vi "mastercontrol.vi"() -> ()   [LabVIEW 2022 SP3]
uses:
  Motion Controllers/NI_controller/-NI_MotionRoutines/MotionSys.ctl
  -ScanSystem/Controls/location.ctl
  Digitizers/-DigitizerRoutines/DigConfig.ctl
  Pulsers/pulser.ctl
  Switch Modules/SwitchOption.ctl
  -ScanSystem/Controls/EKG_Mode.ctl
  Digitizers/-DigitizerRoutines/Digitizer.ctl
  -ScanSystem/Controls/Breath_Mode.ctl
  Spectrometers/OceanOptics/OceanOpticsVIs.llb/SpectrometerType.ctl
  Motion Controllers/-MotionRoutines/MotionGlobals.vi
  Digitizers/-DigitizerRoutines/DigitizerGlobals.vi
  Switch Modules/SwitchGlobals.vi
  Pulsers/PulserGlobals.vi
  <instrlib>/niSwitch/niSwitch.llb/niSwitch Topologies.ctl
  <instrlib>/Newport ESP301/Newport ESP301.lvlib
  <instrlib>/LeCroy Wave Series/LeCroy Wave Series.lvlib
panel:
  in  "Debug Mode?":bool
  in  "Microscopy Scope":refnum<visa-resource-name>="USB0::0x05FF::0x1023::4607N02183::INSTR"
  in  "Initial Setup\nComplete":bool
  in  "Bypass 2nd\nDigi Init":bool
  in  "Breath Trig":T1 items=["Respir Trig Off", "Respir Ring1 (Ch1)", "Respir Ch0", "Dig Edge"]
  in  "Main Digitizer":T2=enum."NI Digitizer"
  in  "EKG Gate":T3 items=["Retro/Prosp Off", "Prosp Ext EKG", "Prosp IQ EKG", "Retro EKG", "Retro IQ", "Retro No EKG"]
  in  "Switch Unit":T4=enum."No Switch"
  in  "Pulser":T5=enum."No Pulser"
  in  "Digitizer Config":T6
  in  "Location":T7
  in  "LeCroy IP Address":refnum<visa-resource-name>="VICP::169.254.24.19"
  in  "Main Spectrometer":T8 items=["No Spectrometer", "Ocean QE_Pro"]
  in  "Select V&A":bool
  in  "Motion System":T9=enum."Galil"
  in  "Start Scan":bool
  in  "Move to Home":bool
  in  "Man Cont":bool
  in  "NI Cards":i32=3
  in  "Therapy":bool
  in  "ExitSendCmd":bool
  # "Motion"
  # "No NI Motion Support!!!!!!!!\nOnly works with 64bit LV."
  # "SCAN"
  # "© 2022\nWeill Cornell"
  # "Options"
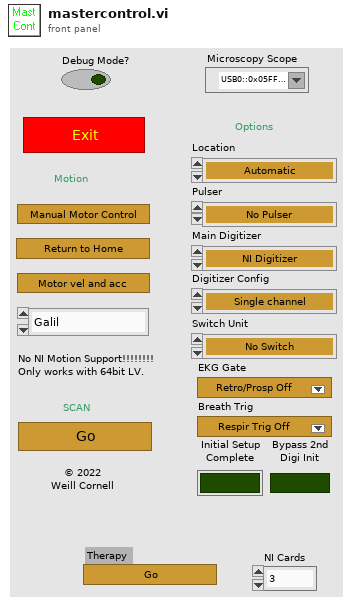
[diagram p1: front panel]
types:
  T1 = typedef "Breath_Mode.ctl" = u16
  T2 = typedef "Digitizer.ctl" = enum16{"Acqiris Digitizer", "NI Digitizer", "LeCroy", "GaGe", "AlazarTech", "No Digitizer", "Teledyne"}
  T3 = typedef "EKG_Mode.ctl" = u16
  T4 = typedef "SwitchOption.ctl" = enum16{"Cytex", "Pickering", "NI Switch", "No Switch", "Riverside USB"}
  T5 = typedef "pulser.ctl" = enum16{"Pan 5900", "Daxsonics", "Agilent 33xxx", "UTEX", "JSR", "WMC Mono-Cycle", "No Pulser", "NYU AVTECH", "Tabor W1281A", "Pan 5800", "Unlisted", "Tabor WX2182B"}
  T6 = typedef "DigConfig.ctl" = enum16{"Single channel", "2 Chans w/ 2 Acqiris", "2 Chans w/ 1 Acqiris", "5-CH Pulser New", "5-CH pulser w/ ann array", "5-pass style ann array", "Empty"}
  T7 = typedef "location.ctl" = enum16{"Automatic", "WCM Main", "Hawaii", "Columbia MM3000", "Columbia  NI System", "NYU", "RRI 2", "UHI Allen", "CUMC RT", "Chiba", "Stony Brook", "WCM Microscopy", "WCM Aeoretch", "WCM Optics Lab", "WCM Main 2Axis", "WCM Rotation", "WCM SAM SMAC", "SERI GP"}
  T8 = typedef "SpectrometerType.ctl" = u16
  T9 = typedef "MotionSys.ctl" = enum16{"MM3000", "NI 735x", "Newport ESP", "No Motion Card", "Galil"}
  T10 = typedef "DigitizerSettings.ctl" = cluster{"Digitizer delay (us) ":dbl, "rf points per line":i32, "lines per plane":i32, "Samp Rate (Hz)":dbl, "Additional dig delay (us)":dbl, "Voltage Scale":dbl, "Pre-Looks":i32, "Offset delay (us)":dbl, "bits A/D":i8, "Avg Num":i32, "DigTimeOut":sgl, "Rel Dig Delay":sgl, "Dig Ch":i32, "LeCroyCluster":cluster{"LeCroy Channels":bool[], "LC read pt offset":dbl, "Sweep Avg":bool}, "Main Digitizer":T2, "Dig Config":T6, "Digitizer ID Cluster":T11, "Trigger Settings":cluster{"Trig Source":u16, "Trig Coupling":u16, "Trig Slope":u16, "Level (mV)":dbl}, "Bulk Acq":bool, "Bulk Start Indexes":i32[], "Data Ref RF":refnum<data-value>, "NI ID/Channel":cluster{"NI ID":refnum<k15>, "NI CH":i32}[], "Total Dig CH":i32, "Xtra Ann Trig delay (us)":dbl, "Fix Z Delay?":bool, "One Way Transmission?":bool, "Data Ref Log":refnum<data-value>}
  T11 = typedef "DigitizerID.ctl" = cluster{"Acqiris/Alazar/SP ID":u32[], "NI Instr Handles":refnum<k15>[], "LeCroy VISA":refnum<visa-resource-name>, "GaGe Handle":cluster{"Handle":u32, "Sample size":u32, "Resolution":i32, "Offset":i32, "Channels":u32, "Boards":u32}, "ATS Ref":string, "Acqiris Address":string[], "ADQRef":refnum<k24>, "adq_cu_ptr":refnum<k24>}
  T12 = typedef "MotionParameters.ctl" = cluster{"No Motion?":bool, "Motion System":T9, "Motion Bd ID":u8, "Motion Profile":string, "# Axis":i8, "Reverse Z axis?":bool, "SMAC Axis":u16, "scan pair":T13, "RT fps":sgl, "Steps per mm":i32[], "Motor Parameters":cluster{"velocity ct/s":dbl[], "accel ct/s^2":dbl[]}, "One Way Scan":bool, "Reverse One Way Scan":bool, "Global Position (mm)":dbl[], "Plane":i32, "Distance between\nscan lines (um)":sgl, "Distance between\nscan planes (um)":sgl, "number of scan planes":i32, "Total steps in line":i32, "Xtra plane\ndistance  (um)":i32, "Xtra planes ":i32, "Add Axis":bool, "overshoot cts":i32, "BKPT Shift":i32, "Scan Start Time (ms)":u32, "ESP VISA":refnum<visa-resource-name>, "3rd Axis":T14, "GL Ref Out":refnum<k7>, "Galil Address":string}
  T13 = typedef "ScanAxis.ctl" = enum16{"y-(x) scan", "x-(y) scan", "z-(x) scan", "z-(y) scan", "y-(z) scan", "x-(z) scan", "w-(x) scan", "w-(y) scan", "w-(z) scan", "x-(w) scan", "y-(w) scan", "z-(w) scan"}
  T14 = typedef "3rdAxis.ctl" = u16
  T15 = enum8{"Enabled", "Disabled", "Disabled and Grayed Out"}
  T16 = enum16{"Absolute Position", "Relative Position", "Velocity", "Relative to Cap Pos", "Modulus Position", "Absolute Contouring", "Relative Contouring"}
  T17 = typedef "niSwitch Topologies.ctl" = string
  T18 = cluster{"Pulser":refnum<vi>, "Switch Unit":refnum<vi>, "Main Digitizer":refnum<vi>, "Digitizer Config":refnum<vi>, "EKG Gate":refnum<vi>, "Breath Trig":refnum<vi>, "Motion System":refnum<vi>, " LeCroy IP Address":refnum<vi>, "Main Spectrometer":refnum<vi>}
  T19 = typedef "Dual XDCR Complete Settings.ctl" = cluster{"Scan Size":dbl[], "XDCR Offset":dbl[], "Found Home":bool, "XDCR Settings":T20[]}
  T20 = typedef "XDCRSettings.ctl" = cluster{"Transducer Name":string, "Motion Settings":cluster{"Distance between\nscan lines (um)":sgl, "Distance between\nscan planes (um)":sgl}, "Digitizer Settings":cluster{"RF data Sampling":cluster{"Sampling Rate":dbl, "Ref Delay (ms)":dbl, "rf points per line":i32}, "Time scale per Div":dbl, "Voltage Scale":dbl, "Additional dig delay (ms)":dbl}, "Filter Prams":cluster{"low cutoff":i32, "order":i32, "high cutoff":i32}, "XDCR Focal Length":dbl, "Data Vertical Center":dbl, "Image Vertical Offset":dbl, "Daxsonics Settings":T21, "Panametrics Settings":T22, "JSR Complete":T23, "UT340 Controls":T38}
  T21 = typedef "Dax_Control_Cluster.ctl" = cluster{"Freq (MHz) ":u16, "Voltage (V)":u16, "Gain (dB)":u16}
  T22 = typedef "Pana5900.ctl" = cluster{"ENERGY (uJ)":u16, "DAMPING (Ohm)":u16, "HP FILT (KHz) ":u16, "LP FILT (MHz)":u16, "MODE":u16, "PRF (KHz)":u16, "GAIN (db)":u16, "COARSE ATTENUATION":u16, "FINE ATTENUATION":u16}
  T23 = typedef "JSR Complete.ctl" = cluster{"JSR Pulse Settings":T24, "JSR Receive Settings":T29, "JSR Trigger Settings":T34}
  T24 = typedef "JSR Pulse.ctl" = cluster{"Damping":T25, "Pulse Energy Level":T26, "Pulser Impedance":T27, "Pulser Voltage (V)":T28}
  T25 = typedef "Damping.ctl" = i16
  T26 = typedef "Energy.ctl" = u16
  T27 = typedef "Z.ctl" = u16
  T28 = typedef "Volt.ctl" = i16
  T29 = typedef "JSR Recieve.ctl" = cluster{"Receiver Mode":T30, "High Pass Filter":T31, "Low Pass Filter":T32, "Gain (dB)":T33}
  T30 = typedef "Mode.ctl" = i8
  T31 = typedef "HPF.ctl" = u16
  T32 = typedef "LPF.ctl" = u16
  T33 = typedef "Gain.ctl" = i8
  T34 = typedef "JSR Trigger.ctl" = cluster{"External Trigger Limit":T35, "Trigger Source":T36, "PRF (Hz)":T37}
  T35 = typedef "Trig Limit.ctl" = i8
  T36 = typedef "Trig Source.ctl" = i8
  T37 = typedef "PRF.ctl" = dbl
  T38 = typedef "UTEX Controls.ctl" = cluster{"High Pass On":bool, "High Pass Filter (MHz)":i16, "Low Pass On":bool, "Low Pass Filter (MHz)":i16, "PE Gain (dB)":i16, "Voltage":i16, "Pulse Width (ns)":dbl, "Mode":bool, "PC Gain (dB)":i16, "Trig Source":bool, "Rep Rate (Hz)":i16, "PULSE":bool}
  T39 = cluster{"Therapy frequency (MHz)":dbl, "Therapy amplitude (mV)":dbl, "time therapy on (s)":dbl, "Therapy Delay (ms) ":dbl, "Time (s)":dbl}
  T40 = cluster{"Handle":u32, "Sample size":u32, "Resolution":i32, "Offset":i32, "Channels":u32, "Boards":u32}
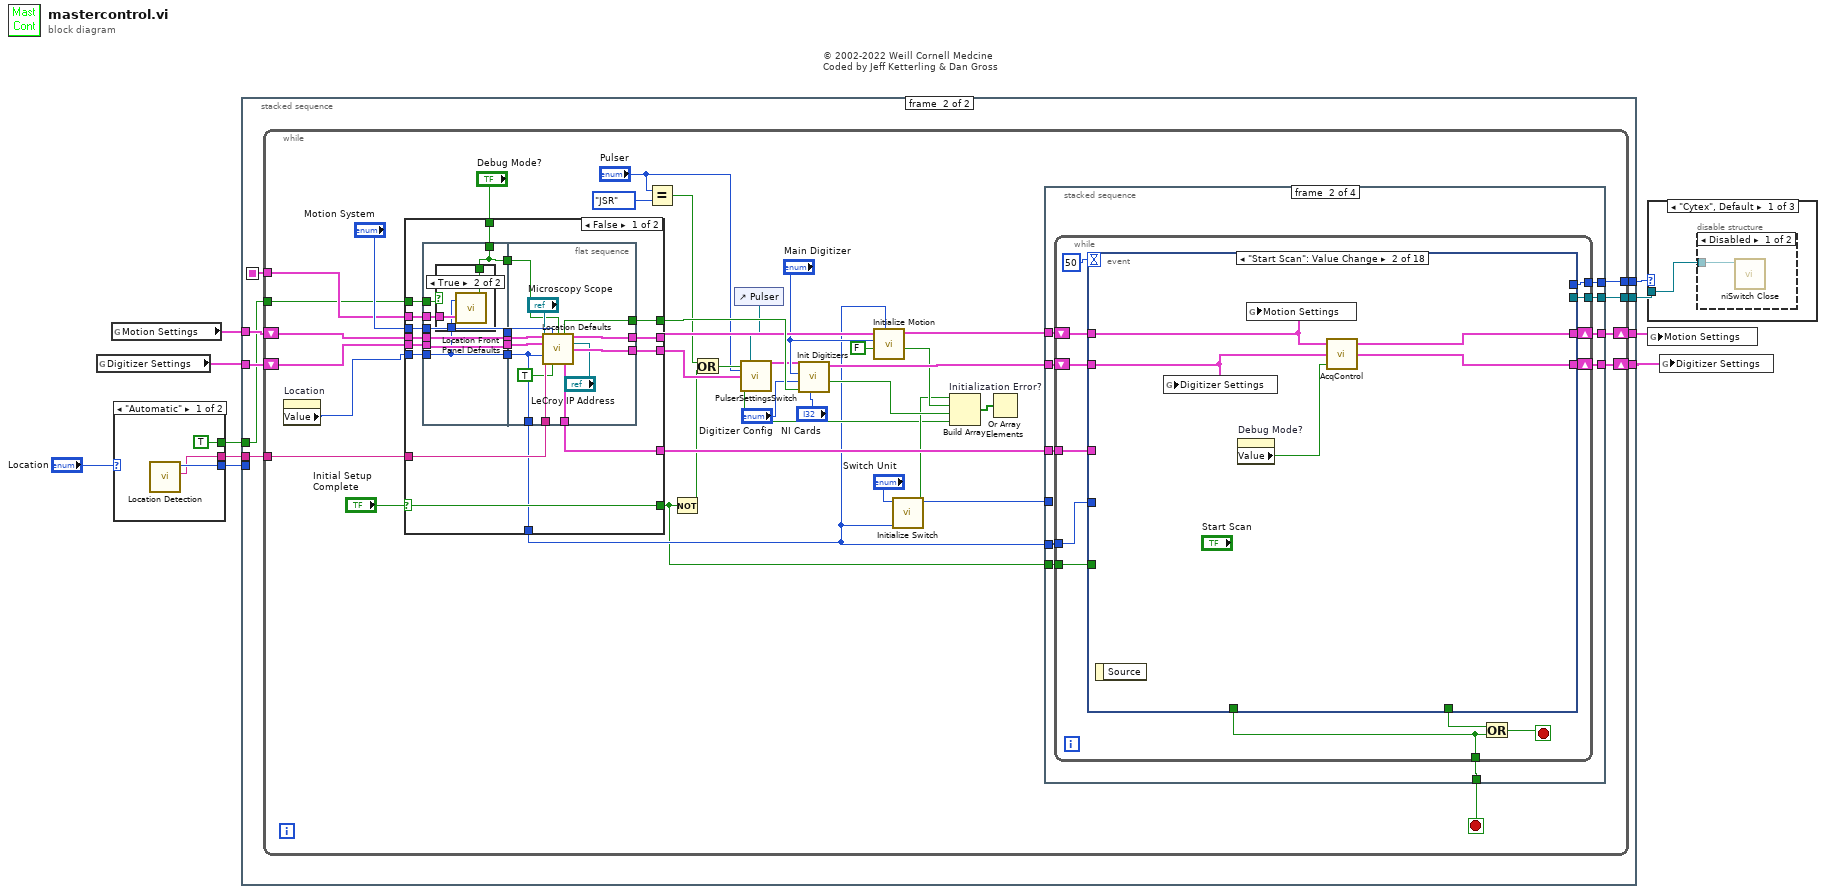
[diagram p0: block diagram]
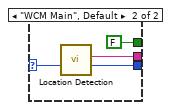
[diagram p2: hidden frame]
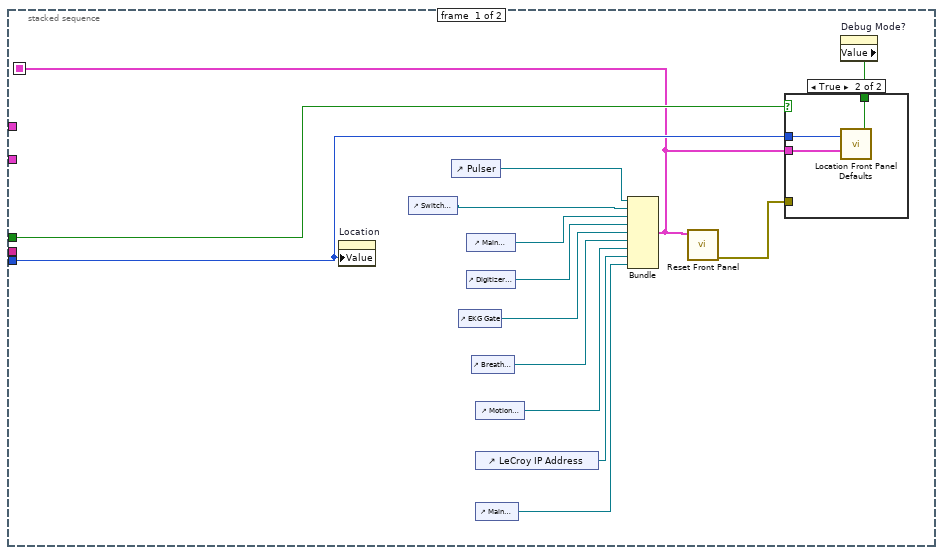
[diagram p3: hidden frame]
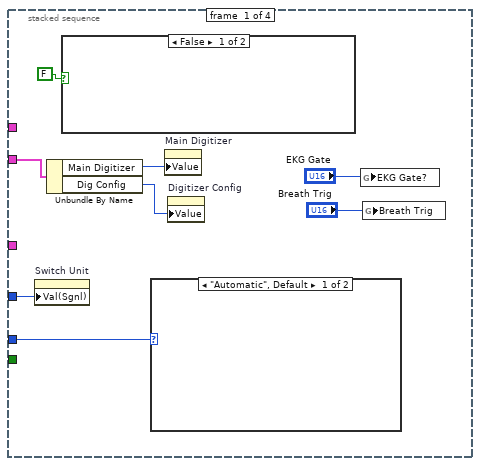
[diagram p5: hidden frame]
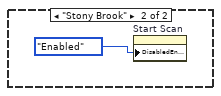
[diagram p6: hidden frame]
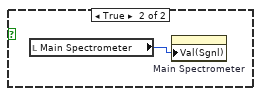
[diagram p7: hidden frame]
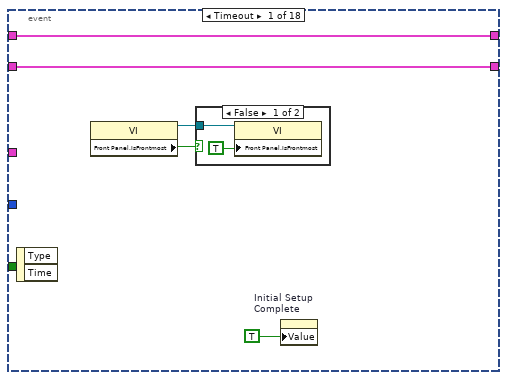
[diagram p8: hidden frame]
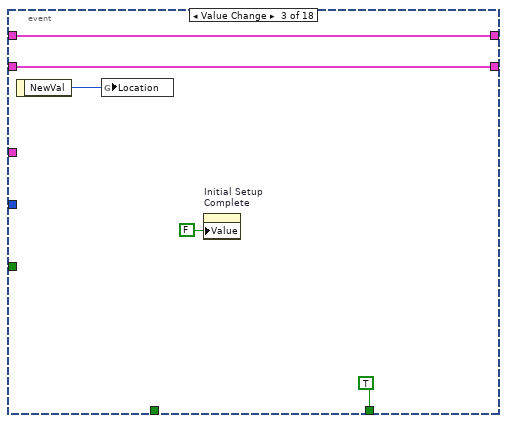
[diagram p10: hidden frame]
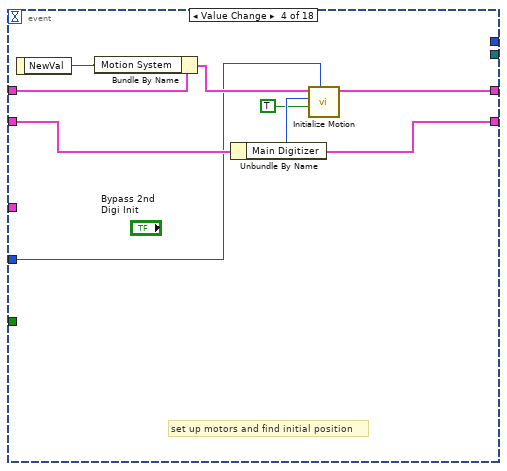
[diagram p11: hidden frame]
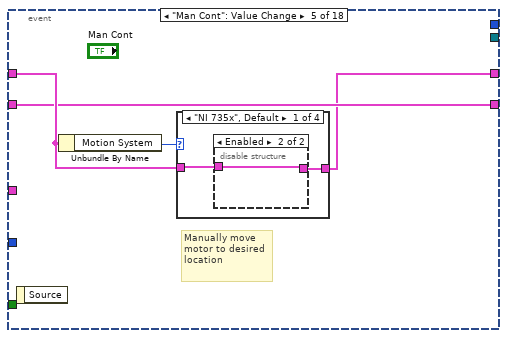
[diagram p12: hidden frame]
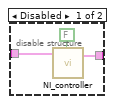
[diagram p13: hidden frame]
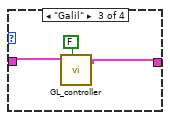
[diagram p15: hidden frame]
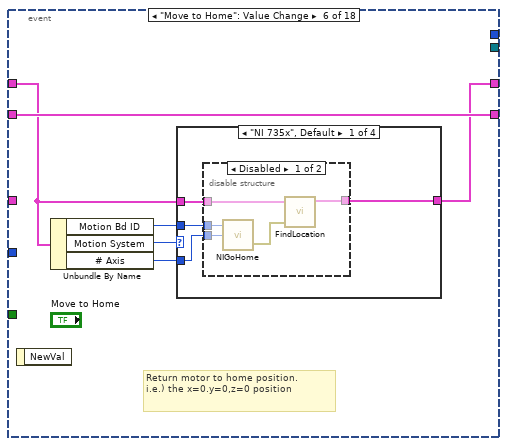
[diagram p17: hidden frame]
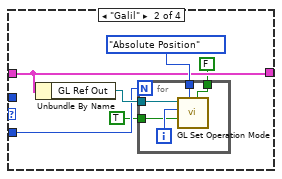
[diagram p19: hidden frame]
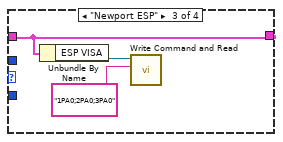
[diagram p20: hidden frame]
diagram:
  # "© 2002-2022 Weill Cornell Medcine\nCoded by Jeff Ketterling & Dan Gross"
  n1 = global read "DigitizerGlobals.vi" "Digitizer Settings"() -> (w6:T10)
  n2 = global read "MotionGlobals.vi" "Motion Settings"() -> (w7:T12)
  n3 = case shown="\"Automatic\"" "Location" {
    selector: "Location" -> [_ w16]
    tunnel: [w13 w16] -> w3
    tunnel: [w12 w14] -> w2
    tunnel: [TRUE ("Load Defaults") FALSE ("Load Defaults")] -> w1
    frame "Automatic" {
      n4 = call "Location Detection.vi"() -> ("Computer Name"=w12:string, "Location"=w13:T7)  [unwired: 10 in]
    }
    frame "WCM Main", Default {
      n5 = call "Location Detection.vi"() -> ("Computer Name"=w14:string)  [unwired: 10 in, 1 out]
    }
  }
  n6 = stacked-sequence {
    seq-local: [w18 _] -> [_ w36]
    tunnel: [_ w42] -> w10
    tunnel: [_ w41] -> w9
    tunnel: [_ w40] -> w5
    tunnel: w6 -> [_ w39]
    tunnel: w7 -> [_ w38]
    tunnel: [_ w37] -> w8
    tunnel: w3 -> [w25 _]
    tunnel: w2 -> [_ w35]
    tunnel: w1 -> [w24 w34]
    frame #0 {
      n7 = property on="Location" class="Enum (strict)"("Value"=w25) -> ()  [unwired: 2 in, 2 out]
      n8 = control-ref of="Switch Unit"() -> (w17:refnum<vi>)
      n9 = control-ref of="Pulser"() -> (w19:refnum<vi>)
      n10 = control-ref of="EKG Gate"() -> (w29:refnum<vi>)
      n11 = control-ref of="Main Digitizer"() -> (w22:refnum<vi>)
      n12 = control-ref of="Digitizer Config"() -> (w23:refnum<vi>)
      n13 = control-ref of="Breath Trig"() -> (w28:refnum<vi>)
      n14 = control-ref of="Motion System"() -> (w27:refnum<vi>)
      n15 = control-ref of="LeCroy IP Address"() -> (w26:refnum<vi>)
      n16 = control-ref of="Main Spectrometer"() -> (w30:refnum<vi>)
      n17 = Bundle("Pulser"=w19, "Switch Unit"=w17, "Main Digitizer"=w22, "Digitizer Config"=w23, "EKG Gate"=w29, "Breath Trig"=w28, "Motion System"=w27, "LeCroy IP Address"=w26, "Main Spectrometer"=w30) -> (w18:T18)  [unwired: 1 in]
      n18 = call "Reset Front Panel.vi"("output cluster"=w18) -> ("error out"=w20:errorcluster)  [unwired: 10 in]
      n19 = property on="Debug Mode?" class="Bool (strict)"() -> ("Value"=w21:bool)  [unwired: 2 in, 2 out]
      n20 = case shown="True" w24 {
        tunnel: w18 -> [_ w32]
        tunnel: w25 -> [_ w33]
        tunnel: w21 -> [_ w31]
        tunnel: w20 -> [_ _]
        frame False {
        }
        frame True {
          n21 = call "Location Front Panel Defaults.vi"("Debug Mode?"=w31, "output cluster"=w32, "Location"=w33) -> ()
        }
      }
    }
    frame #1 {
      n22 = while {
        tunnel: [w81] -> w42
        tunnel: [w80] -> w41
        shift-right: [w79] -> w40
        shift-left: w39 -> [w76]
        shift-right: [w78] -> w37
        shift-left: w38 -> [w77]
        tunnel: w36 -> [w60]
        tunnel: w35 -> [w58]
        tunnel: w34 -> [w57]
        stop <- w82 stop-if-true
        n23 = property on="Location" class="Enum (strict)"() -> ("Value"=w43:T7)  [unwired: 2 in, 2 out]
        n24 = case shown="False" "Initial Setup\nComplete" {
          selector: "Initial Setup\nComplete" -> [w338 w381]
          tunnel: w77 -> [w353 w379]
          tunnel: [w352 w377] -> w70
          tunnel: w76 -> [w351 w384]
          tunnel: [w341 w384] -> w73
          tunnel: [w350 w383] -> w74
          tunnel: w43 -> [w347 w380]
          tunnel: [w349 w382] -> w75
          tunnel: "Motion System" -> [w348 w378]
          tunnel: w60 -> [w342 _]
          tunnel: w58 -> [w340 _]
          tunnel: w57 -> [w339 _]
          tunnel: [w338 w381] -> w44
          tunnel: "Debug Mode?" -> [w337 _]
          tunnel: [w336 w380] -> w45
          frame False {
            n25 = flat-sequence {
              tunnel: w347 -> [w356]
              tunnel: w348 -> [w358]
              tunnel: w351 -> [w359]
              tunnel: w353 -> [w360]
              tunnel: [w360] -> w346
              tunnel: [w359] -> w345
              tunnel: [w358] -> w344
              tunnel: [w356] -> w343
              tunnel: w342 -> [w357]
              tunnel: w339 -> [w355]
              tunnel: w337 -> [w354]
              tunnel: [w354] -> w335
              tunnel: [w375] -> w352
              tunnel: [w370] -> w350
              tunnel: [w373] -> w349
              tunnel: w346 -> [w376]
              tunnel: w345 -> [w374]
              tunnel: w344 -> [w372]
              tunnel: w343 -> [w366]
              tunnel: [w371] -> w341
              tunnel: w340 -> [w369]
              tunnel: [w366] -> w336
              tunnel: w335 -> [w364]
              frame #0 {
                n26 = case shown="True" w355 {
                  tunnel: w357 -> [_ w363]
                  tunnel: w356 -> [_ w361]
                  tunnel: w354 -> [_ w362]
                  frame False {
                  }
                  frame True {
                    n27 = call "Location Front Panel Defaults.vi"("Debug Mode?"=w362, "output cluster"=w363, "Location"=w361) -> ()
                  }
                }
              }
              frame #1 {
                n28 = call "Location Defaults.vi"("Motion Settings In"=w376, "Motion System"=w372, "Debug Mode?"=w364, "Digitizer Settings In"=w374, "LeCroy IP Address"="LeCroy IP Address", "Microscopy Scope"="Microscopy Scope", "Location In"=w366, "Computer Name"=w369, "Create Data Folder"=TRUE) -> ("Bypass 2nd dig init"=w370:bool, "Motion Settings"=w375:T12, "Digitizer Settings"=w371:T10, "Dual XDCR Settings"=w373:T19)  [unwired: 1 in, 2 out]
              }
            }
          }
          frame True {
            n29 = global read "SwitchGlobals.vi" "Dual XDCR Settings"() -> (w382:T19)
            n30 = Bundle By Name(cluster=w379, "Motion System"=w378) -> (w377:T12)
            n31 = property on="Bypass 2nd\nDigi Init" class="Bool (strict)"() -> ("Value"=w383:bool)  [unwired: 2 in, 2 out]
          }
        }
        n32 = Equal?(x="Pulser", y=pulser."JSR") -> (x = y?=w48:bool)
        n33 = Not(x=w44) -> (.not. x?=w47:bool)
        n34 = Or(x=w48, y=w47) -> (x .or. y?=w51:bool)
        n35 = control-ref of="Pulser"() -> (w46:refnum<vi>)
        n36 = call "PulserSettingsSwitch.vi"("Initilize?"=w51, "Pulser Ref"=w46, "Pulser"="Pulser", "Digitizer Settings in"=w73) -> ("Digitizer Settings out"=w55:T10, "Initialization Failed!!"=w54:bool)  [unwired: 9 in, 1 out]
        n37 = call "Init Digitizers.vi"("NI Cards"="NI Cards", "Bypass 2nd Digitizer Init"=w74, "Digitizer Config"="Digitizer Config", "Main Digitizer"="Main Digitizer", "Digitizer Settings in"=w55) -> ("Initialization Failed!!"=w65:bool, "Digitizer Settings"=w68:T10)  [unwired: 4 in, 1 out]
        n38 = call "Initialize Motion.vi"("Location"=w45, "Bypass Motion Init"=FALSE, "Main Digitizer"="Main Digitizer", "Motion Settings In"=w70) -> ("Initialization Failed!!"=w66:bool, "Motion Settings"=w69:T12)  [unwired: 5 in, 1 out]
        n39 = call "Initialize Switch.vi"("Location"=w45, "Switch Unit In"="Switch Unit") -> ("Initialization Failed!!"=w62:bool, "Switch Unit"=w63:T4)  [unwired: 8 in]
        n40 = Build Array "Initialization Error?"(w62, w66, w65, w54) -> (w67:bool[])
        n41 = Or Array Elements(Boolean array=w67) -> ()  [unwired: 1 out]
        n42 = stacked-sequence {
          tunnel: [_ w98 _ _] -> w80
          tunnel: [_ w97 _ _] -> w81
          tunnel: [_ w93 _ _] -> w82
          tunnel: w68 -> [w86 w96 _ w302]
          tunnel: [_ w102 _ _] -> w79
          tunnel: w69 -> [_ w99 _ w303]
          tunnel: [_ w101 _ _] -> w78
          tunnel: w75 -> [_ w100 _ _]
          tunnel: w63 -> [w87 _ _ _]
          tunnel: w45 -> [w83 w95 _ _]
          tunnel: w44 -> [_ w94 _ _]
          frame #0 {
            n43 = property on="Switch Unit" class="Enum (strict)"("Val(Sgnl)"=w87) -> ()  [unwired: 2 in, 2 out]
            n44 = Unbundle By Name(w86) -> ("Main Digitizer"=w85:T2, "Dig Config"=w84:T6)
            n45 = case shown="False" FALSE {
              frame False {
              }
              frame True {
                n46 = local read "Main Spectrometer"() -> (w92:T8)
                n47 = property on="Main Spectrometer" class="Ring (strict)"("Val(Sgnl)"=w92) -> ()  [unwired: 2 in, 2 out]
              }
            }
            n48 = case shown="\"Automatic\", Default" w83 {
              frame "Automatic", Default {
              }
              frame "Stony Brook" {
                n49 = property on="Start Scan" class="Bool"("DisabledEnum"=T15."Enabled" ("Disabled")) -> ()  [unwired: 2 in, 2 out]
              }
            }
            n50 = property on="Main Digitizer" class="Enum (strict)"("Value"=w85) -> ()  [unwired: 2 in, 2 out]
            n51 = property on="Digitizer Config" class="Enum (strict)"("Value"=w84) -> ()  [unwired: 2 in, 2 out]
            n52 = global write "MotionGlobals.vi" "EKG Gate?"("EKG Gate") -> ()
            n53 = global write "MotionGlobals.vi" "Breath Trig"("Breath Trig") -> ()
          }
          frame #1 {
            n54 = while {
              shift-right: [w111] -> w102
              shift-left: w96 -> [w112]
              shift-right: [w109] -> w101
              shift-left: w99 -> [w110]
              tunnel: w100 -> [w108]
              tunnel: [w107] -> w98
              tunnel: [w106] -> w97
              tunnel: w95 -> [w105]
              tunnel: w94 -> [w104]
              tunnel: [w103] -> w93
              stop <- w114 stop-if-true
              n55 = event shown="[1] \"Start Scan\": Value Change" {
                selector: _ -> [_ _ _ _ _ _ _ _ _ _ _ _ _ _ _ _ _ _]
                dyn-events: _ -> [_ _ _ _ _ _ _ _ _ _ _ _ _ _ _ _ _ _]
                timeout: 50 -> [_ _ _ _ _ _ _ _ _ _ _ _ _ _ _ _ _ _]
                tunnel: [_ _ TRUE _ _ _ _ _ _ TRUE TRUE TRUE TRUE _ _ TRUE _ _] -> w113
                tunnel: w112 -> [w120 w124 w131 w136 w142 w162 w191 w210 w248 w255 w261 w264 w268 w270 w273 w279 w286 w288]
                tunnel: [w120 w125 w131 w136 w142 w162 w191 w208 w248 w254 w261 w264 w268 w270 w273 w278 w286 w288] -> w111
                tunnel: w110 -> [w119 w127 w130 w138 w143 w159 w189 w209 w247 w252 w260 w263 w267 w269 w272 w276 w285 w287]
                tunnel: [w119 w126 w130 w139 w141 w157 w188 w207 w247 w252 w260 w263 w267 w269 w272 w276 w285 w287] -> w109
                tunnel: w108 -> [_ _ _ _ _ _ _ w206 _ _ _ _ _ _ _ _ _ _]
                tunnel: [_ _ _ _ _ _ _ w205 _ _ _ _ _ _ _ _ _ _] -> w107
                tunnel: [_ _ _ _ _ _ _ w203 _ _ _ _ _ _ _ _ _ _] -> w106
                tunnel: w105 -> [_ _ _ w133 _ _ w187 w204 _ _ _ _ _ _ _ _ _ _]
                tunnel: w104 -> [_ _ _ _ _ _ _ w202 _ _ _ _ _ _ _ _ _ _]
                tunnel: [_ _ _ _ _ _ _ _ "ExitSendCmd" _ _ _ _ _ _ _ _ _] -> w103
                event Timeout {
                  n56 = event-data() -> ()  [unwired: 3 out]
                  n57 = property class="VI"() -> (reference out=w118:refnum<vi>, "Front Panel.IsFrontmost"=w117:bool)  [unwired: 2 in, 1 out]
                  n58 = case shown="False" w117 {
                    tunnel: w118 -> [w122 _]
                    frame False {
                      n59 = property class="VI"(reference=w122, "Front Panel.IsFrontmost"=TRUE) -> ()  [unwired: 1 in, 2 out]
                    }
                    frame True {
                    }
                  }
                  n60 = property on="Initial Setup\nComplete" class="Bool (strict)"("Value"=TRUE ("Initial Setup\nComplete")) -> ()  [unwired: 2 in, 2 out]
                }
                event "Start Scan": Value Change {
                  n61 = event-data() -> ()  [unwired: 2 out]
                  n62 = global write "DigitizerGlobals.vi" "Digitizer Settings"(w124) -> ()
                  n63 = property on="Debug Mode?" class="Bool (strict)"() -> ("Value"=w123:bool)  [unwired: 2 in, 2 out]
                  n64 = global write "MotionGlobals.vi" "Motion Settings"(w127) -> ()
                  n65 = call "AcqControl.vi"("Debug Mode?"=w123, "Digitizer Settings"=w124, "Motion Settings In"=w127) -> ("Digitizer Settings Out"=w125:T10, "Motion Settings Out"=w126:T12)  [unwired: 1 in]
                }
                event Value Change {
                  n66 = event-data() -> ("NewVal"=w129:T7)  [unwired: 1 out]
                  n67 = global write "MotionGlobals.vi" "Location"(w129) -> ()
                  n68 = property on="Initial Setup\nComplete" class="Bool (strict)"("Value"=FALSE ("Initial Setup\nComplete")) -> ()  [unwired: 2 in, 2 out]
                }
                event Value Change {
                  # "set up motors and find initial position"
                  n69 = event-data() -> ("NewVal"=w140:T9)  [unwired: 1 out]
                  n70 = Bundle By Name(cluster=w138, "Motion System"=w140) -> (w137:T12)
                  n71 = Unbundle By Name(w136) -> ("Main Digitizer"=w135:T2)
                  n72 = call "Initialize Motion.vi"("Location"=w133, "Bypass Motion Init"=TRUE, "Main Digitizer"=w135, "Motion Settings In"=w137) -> ("Motion Settings"=w139:T12)  [unwired: 5 in, 2 out]
                }
                event "Man Cont": Value Change {
                  # "Manually move motor to desired\nlocation"
                  n73 = event-data() -> ()  [unwired: 2 out]
                  n74 = Unbundle By Name(w143) -> ("Motion System"=w144:T9)
                  n75 = case shown="\"NI 735x\", Default" w144 {
                    tunnel: w143 -> [w146 w152 w155 w156]
                    tunnel: [w145 w151 w154 w156] -> w141
                    frame "NI 735x", Default {
                      n76 = disable-structure shown="Enabled" {
                        disable-tunnel: w146 -> [w148 w150]
                        disable-tunnel: [w147 w150] -> w145
                        frame Disabled {
                          n77 = call "NI_controller.VI"("Motion Settings"=w148, "Initialize"=FALSE) -> ("Motion Settings Out"=w147:T12)  [unwired: 3 in, 1 out]
                        }
                        frame Enabled {
                        }
                      }
                    }
                    frame "Newport ESP" {
                      n78 = call "ESPControl.vi"("Motion Settings"=w152) -> ("Motion Settings Out"=w151:T12)  [unwired: 4 in, 1 out]
                    }
                    frame "Galil" {
                      n79 = call "GL_controller.VI"("Motion Settings"=w155, "Initialize"=FALSE) -> ("Motion Settings Out"=w154:T12)  [unwired: 3 in, 1 out]
                    }
                    frame "No Motion Card" {
                    }
                  }
                }
                event "Move to Home": Value Change {
                  # "Return motor to home position.\ni.e.) the x=0.y=0,z=0 position"
                  n80 = event-data() -> ()  [unwired: 2 out]
                  n81 = Unbundle By Name(w159) -> ("Motion Bd ID"=w161:u8, "Motion System"=w160:T9, "# Axis"=w158:i8)
                  n82 = case shown="\"NI 735x\", Default" w160 {
                    tunnel: w161 -> [w166 _ _ _]
                    tunnel: w159 -> [w164 w176 w183 w186]
                    tunnel: w158 -> [w165 w174 _ _]
                    tunnel: [w163 w176 w183 w186] -> w157
                    frame "NI 735x", Default {
                      n83 = disable-structure shown="Disabled" {
                        disable-tunnel: w166 -> [w171 _]
                        disable-tunnel: w165 -> [w170 _]
                        disable-tunnel: w164 -> [w168 _]
                        disable-tunnel: [w167 _] -> w163
                        frame Disabled {
                          n84 = call "NIGoHome.vi"("# Axis"=w170, "Board ID"=w171) -> ("error out"=w169:errorcluster)  [unwired: 1 in, 1 out]
                          n85 = call "FindLocation.vi"("Motion Settings"=w168, "error in (no error)"=w169) -> ("Motion Settings Out"=w167:T12)  [unwired: 1 in, 3 out]
                        }
                        frame Enabled {
                        }
                      }
                    }
                    frame "Galil" {
                      n86 = Unbundle By Name(w176) -> ("GL Ref Out"=w175:refnum<k7>)
                      n87 = for {
                        N: w174 -> [_]
                        tunnel: T16."Absolute Position" ("Position Mode (Absolute)") -> [w182]
                        tunnel: w175 -> [w181]
                        tunnel: TRUE ("Start Now?") -> [w179]
                        tunnel: FALSE ("LimitWarning?") -> [w178]
                        i -> [w180]
                        n88 = call "GL Set Operation Mode.vi"("LimitWarning?"=w178, "Position Mode (Absolute)"=w182, "Start Now?"=w179, "Axis"=w180, "Galil.IGalil"=w181) -> ()  [unwired: 4 in, 3 out]
                      }
                    }
                    frame "Newport ESP" {
                      n89 = Unbundle By Name(w183) -> ("ESP VISA"=w184:refnum<visa-resource-name>)
                      n90 = call <instrlib>:"Write Command and Read.vi"("Command"="1PA0;2PA0;3PA0", "VISA resource name"=w184) -> ()  [unwired: 5 in, 3 out]
                    }
                    frame "No Motion Card" {
                    }
                  }
                }
                event "Select V&A": Value Change {
                  # "Need to set global Motor Parameters\nto default for velocity and accel"
                  n91 = event-data() -> ()  [unwired: 2 out]
                  n92 = Unbundle By Name(w189) -> ("Motion System"=w190:T9)
                  n93 = case shown="\"NI 735x\", Default" w190 {
                    tunnel: w189 -> [w196 w198 w201]
                    tunnel: [w195 w199 w200] -> w188
                    tunnel: w187 -> [w194 _ _]
                    frame "NI 735x", Default {
                      n94 = call "UpdateVandAGlobals.vi"("Motion Settings"=w196) -> ("Motion Settings Out"=w195:T12)  [unwired: 3 in, 1 out]
                      n95 = call "Initialize_NI.vi"("Motion Settings"=w195, "Bypass Motion Init"=TRUE ("Bypass Init"), "Location"=w194) -> ()  [unwired: 2 in, 3 out]
                    }
                    frame "Galil" {
                      n96 = Unbundle By Name(w198) -> ("GL Ref Out"=w197:refnum<k7>)
                      n97 = call "GL_SetVandA.vi"("Motion Settings"=w198, "Refnum in"=w197) -> ("Motion Settings Out"=w199:T12)  [unwired: 7 in, 2 out]
                    }
                    frame "Newport ESP" {
                      n98 = call "UpdateVandAGlobals.vi"("Motion Settings"=w201) -> ("Motion Settings Out"=w200:T12)  [unwired: 3 in, 1 out]
                      n99 = call "Init ESP.vi"("Motion Settings In"=w200) -> ()  [unwired: 11 in]
                    }
                  }
                  n100 = local write "Select V&A"(FALSE) -> ()
                }
                event Value Change {
                  n101 = event-data() -> ("NewVal"=w203:T4)  [unwired: 1 out]
                  n102 = case shown="\"NI Switch\"" w203 {
                    tunnel: [_ w215 _ _] -> w205
                    tunnel: w209 -> [w211 w214 w221 w231]
                    tunnel: [w211 w214 w221 w228] -> w207
                    tunnel: w210 -> [w212 w213 w220 w230]
                    tunnel: [w212 w213 w220 w229] -> w208
                    tunnel: w206 -> [_ _ _ w224]
                    tunnel: w204 -> [_ _ _ w227]
                    tunnel: w202 -> [_ _ _ w226]
                    frame "Pickering" {
                    }
                    frame "NI Switch" {
                      n103 = disable-structure shown="Disabled" {
                        disable-tunnel: [w219 _] -> w215
                        frame Disabled {
                          n104 = call <instrlib>:"niSwitch Initialize With Topology.vi"("reset device (boolean value)"=TRUE, "topology name"=T17 "2593/16x1 Mux", "resource name"=refnum<k15> "NISwitch") -> ("instrument handle out"=w219:refnum<k15>)  [unwired: 7 in, 1 out]
                          n105 = global write "MotionGlobals.vi" "NI Switch"(w219) -> ()
                        }
                        frame Enabled {
                        }
                      }
                    }
                    frame "No Switch", Default {
                    }
                    frame "Riverside USB" {
                      n106 = Unbundle By Name(w224) -> ("XDCR Settings"=w223:T20[])
                      n107 = Array Size(array=w223) -> (size(s)=w225:i32)
                      n108 = Not Equal To 0?(x=w225) -> (x != 0?=w222:bool)
                      n109 = case shown="True" w222 {
                        tunnel: w231 -> [w233 w244]
                        tunnel: w230 -> [w232 w243]
                        tunnel: [w232 w242] -> w229
                        tunnel: w224 -> [_ w241]
                        tunnel: [w233 w239] -> w228
                        tunnel: w227 -> [_ w238]
                        tunnel: w226 -> [_ w236]
                        frame False {
                        }
                        frame True {
                          n110 = property on="Pulser" class="Enum (strict)"() -> ("Value"=w235:T5)  [unwired: 2 in, 2 out]
                          n111 = property on="Debug Mode?" class="Bool (strict)"() -> ("Value"=w234:bool)  [unwired: 2 in, 2 out]
                          n112 = call "SetupXDCRDefaults.vi"("Digitizer Settings in"=w243, "Pulser"=w235, "Debug Mode?"=w234, "Motion Settings in"=w244, "Dual XDCR Settings In"=w241, "Location"=w238, "Initial Setup Complete"=w236) -> ("Digitizer Settings out"=w242:T10, "Motion Settings out"=w240:T12, "Dual XDCR Settings"=w237:T19)  [unwired: 3 in, 3 out]
                          n113 = global write "SwitchGlobals.vi" "Dual XDCR Settings"(w237) -> ()
                          n114 = call "FindLocation.vi"("Motion Settings"=w240) -> ("Motion Settings Out"=w239:T12)  [unwired: 2 in, 3 out]
                        }
                      }
                    }
                  }
                  n115 = global write "SwitchGlobals.vi" "Switch Unit"(w203) -> ()
                }
                event "ExitSendCmd": Value Change {
                  n116 = event-data() -> ()  [unwired: 5 out]
                  n117 = property on="Pulser" class="Enum (strict)"() -> ("Value"=w246:T5)  [unwired: 2 in, 2 out]
                  n118 = case shown="\"Pan 5900\", Default" w246 {
                    frame "Pan 5900", Default {
                    }
                    frame "JSR" {
                      n119 = global read "PulserGlobals.vi" "JSR VISA"() -> (w250:refnum<visa-resource-name>)
                      n120 = property on="Initial Setup\nComplete" class="Bool (strict)"("Value"=FALSE ("Initial Setup\nComplete")) -> ()  [unwired: 2 in, 2 out]
                      n121 = call <instrlib>:"dpr300 Close.vi"("VISA resource name"=w250) -> ()  [unwired: 10 in, 1 out]
                    }
                  }
                }
                event Value Change {
                  n122 = event-data() -> ("NewVal"=w253:T6)  [unwired: 1 out]
                  n123 = Bundle By Name(cluster=w255, "Dig Config"=w253) -> (w254:T10)
                  n124 = property on="Initial Setup\nComplete" class="Bool (strict)"("Value"=FALSE ("Initial Setup\nComplete")) -> ()  [unwired: 2 in, 2 out]
                }
                event Value Change {
                  n125 = event-data() -> ("NewVal"=w259:T5)  [unwired: 1 out]
                  n126 = global write "PulserGlobals.vi" "Pulser"(w259) -> ()
                  n127 = property on="Initial Setup\nComplete" class="Bool (strict)"("Value"=FALSE ("Initial Setup\nComplete")) -> ()  [unwired: 2 in, 2 out]
                }
                event "Initial Setup\nComplete": Value Change {
                  n128 = event-data() -> ()  [unwired: 2 out]
                }
                event "Debug Mode?": Value Change {
                  n129 = event-data() -> ()  [unwired: 2 out]
                  n130 = property on="Initial Setup\nComplete" class="Bool (strict)"("Value"=FALSE ("Initial Setup\nComplete")) -> ()  [unwired: 2 in, 2 out]
                }
                event Value Change {
                  n131 = event-data() -> ("NewVal"=w271:T3)  [unwired: 1 out]
                  n132 = global write "MotionGlobals.vi" "EKG Gate?"(w271) -> ()
                }
                event Value Change {
                  n133 = event-data() -> ("NewVal"=w274:T1)  [unwired: 1 out]
                  n134 = global write "MotionGlobals.vi" "Breath Trig"(w274) -> ()
                }
                event Value Change {
                  n135 = event-data() -> ("NewVal"=w277:T2)  [unwired: 1 out]
                  n136 = Bundle By Name(cluster=w279, "Main Digitizer"=w277) -> (w278:T10)
                  n137 = property on="Initial Setup\nComplete" class="Bool (strict)"("Value"=FALSE ("Initial Setup\nComplete")) -> ()  [unwired: 2 in, 2 out]
                }
                event "Therapy": Value Change {
                  # "Therapy solo"
                  n138 = event-data() -> ()  [unwired: 2 out]
                  n139 = global read "PulserGlobals.vi" "Therapy Settings"() -> (w284:T39)
                  n140 = Unbundle By Name(w284) -> ("Therapy frequency (MHz)"=w283:dbl, "Therapy amplitude (mV)"=w282:dbl, "time therapy on (s)"=w281:dbl)
                  n141 = call "Therapy.vi"("Theraputic Freq (MHz)"=w283, "Time on"=w281, "Therapy amplitude (mV)"=w282) -> ()  [unwired: 3 in, 3 out]
                }
                event Value Change {
                  n142 = event-data() -> ("OldVal"=w289:T8, "NewVal"=w290:T8)  [unwired: 1 out]
                  n143 = global write "MotionGlobals.vi" "Main Spectrometer"(w290) -> ()
                  n144 = case shown="0, Default" w290 {
                    tunnel: w289 -> [w291 _]
                    frame 0, Default {
                      n145 = case shown="1" w291 {
                        tunnel: [_ w292] -> _
                        frame 0, Default {
                        }
                        frame 1 {
                          # "OceanLVClose"
                          n146 = global read "MotionGlobals.vi" "Ocean Wrapper"() -> (w292:u32)
                        }
                      }
                    }
                    frame 1 {
                      # "OceanLVInit"
                    }
                  }
                }
              }
              n147 = Or(x=w113, y=w103) -> (x .or. y?=w114:bool)
            }
          }
          frame #2 {
            # "Delete local temp files"
            n148 = global read "MotionGlobals.vi" "TempPath"() -> (w293:path)
            n149 = List Folder(path=w293) -> (path out=w295:path, filenames=w294:string[], error out=w296:errorcluster)  [unwired: 1 in, 3 out]
            n150 = case shown="No Error" w296 {
              tunnel: w295 -> [w298 _]
              tunnel: w294 -> [w297 _]
              frame No Error {
                n151 = for {
                  tunnel: w298 -> [w300]
                  tunnel: w297 -> [w299] mode=indexing
                  n152 = Build Path(base path=w300, name or relative path=w299) -> (appended path=w301:path)
                  n153 = Delete(path (use dialog)=w301) -> ()  [unwired: 1 in, 6 out]
                }
              }
              frame Error {
              }
            }
          }
          frame #3 {
            n154 = Unbundle By Name(w303) -> ("Motion System"=w304:T9, "# Axis"=w305:i8)
            n155 = Unbundle By Name(w302) -> ("Main Digitizer"=w306:T2)
            n156 = case shown="\"NI 735x\", Default" w304 {
              tunnel: w305 -> [_ w324 _]
              tunnel: w303 -> [_ w323 w334]
              frame "NI 735x", Default {
              }
              frame "Newport ESP" {
                n157 = Unbundle By Name(w323) -> ("ESP VISA"=w322:refnum<visa-resource-name>)
                n158 = for {
                  N: w324 -> [_]
                  tunnel: w322 -> [w329]
                  tunnel: [w328] -> w326
                  tunnel: [w327] -> w325
                  i -> [w331]
                  n159 = Increment(x=w331) -> (x+1=w332:i32)
                  n160 = call <instrlib>:"Enable Disable Motor.vi"("Action (OFF)"=FALSE, "Axis (1)"=w332, "VISA resource name"=w329) -> ("error out"=w327:errorcluster, "VISA resource name out"=w328:refnum<visa-resource-name>)  [unwired: 3 in]
                }
                n161 = call <instrlib>:"Close.vi"("error in (no error)"=w325, "VISA resource name"=w326) -> ()  [unwired: 9 in, 1 out]
              }
              frame "Galil" {
                n162 = Unbundle By Name(w334) -> ("GL Ref Out"=w333:refnum<k7>)
                n163 = Close Reference(reference=w333) -> ()  [unwired: 1 in, 1 out]
              }
            }
            n164 = case shown="\"NI Digitizer\"" w306 {
              tunnel: w302 -> [_ w310 w313 w318 _ w321]
              frame "Acqiris Digitizer", Default {
              }
              frame "NI Digitizer" {
                n165 = Unbundle By Name(w310) -> ("Digitizer ID Cluster.NI Instr Handles"=w309:refnum<k15>[])
                n166 = for {
                  tunnel: w309 -> [w311] mode=indexing
                  n167 = call <instrlib>:"niScope Close.vi"("instrument handle"=w311) -> ()  [unwired: 1 in, 14 out]
                }
              }
              frame "LeCroy" {
                n168 = Unbundle By Name(w313) -> ("Digitizer ID Cluster.LeCroy VISA"=w312:refnum<visa-resource-name>)
                n169 = call <instrlib>:"Write.vi"("Write Buffer"="VBS 'app.acquisition.Horizontal.HorOffsetOrigin=5'", "VISA resource name"=w312) -> ("error out"=w314:errorcluster, "VISA resource name out"=w315:refnum<visa-resource-name>)  [unwired: 7 in, 1 out]
                n170 = call <instrlib>:"Close.vi"("error in (no error)"=w314, "VISA resource name"=w315) -> ()  [unwired: 9 in, 1 out]
              }
              frame "GaGe" {
                n171 = Unbundle By Name(w318) -> ("Digitizer ID Cluster.GaGe Handle"=w317:T40)
                n172 = call "CsTool-FreeSystemFill.vi"("Handle Cluster"=w317) -> ()  [unwired: 1 out]
              }
              frame "AlazarTech" {
              }
              frame "Teledyne" {
                n173 = Unbundle By Name(w321) -> ("Digitizer ID Cluster.ADQRef"=w320:refnum<k24>, "Digitizer ID Cluster.adq_cu_ptr"=w319:refnum<k24>)
                n174 = call "SPADQ_DeleteControlUnit.vi"("adq_cu_ptr"=w319, "ADQAPI Ref"=w320) -> ()  [unwired: 9 in, 1 out]
              }
            }
            n175 = case shown="0, Default" "Main Spectrometer" {
              tunnel: [_ w308] -> _
              frame 0, Default {
              }
              frame 1 {
                # "OceanLVClose"
                n176 = global read "MotionGlobals.vi" "Ocean Wrapper"() -> (w308:u32)
              }
            }
          }
        }
      }
    }
  }
  n177 = case shown="\"Cytex\", Default" w10 {
    tunnel: w9 -> [w385 _ _]
    frame "Cytex", Default {
      n178 = disable-structure shown="Disabled" {
        disable-tunnel: w385 -> [w386 _]
        frame Disabled {
          n179 = call <instrlib>:"niSwitch Close.vi"("instrument handle"=w386) -> ()  [unwired: 10 in, 1 out]
        }
        frame Enabled {
        }
      }
    }
    frame "Pickering" {
    }
    frame "NI Switch" {
    }
  }
  n180 = global write "MotionGlobals.vi" "Motion Settings"(w8) -> ()
  n181 = global write "DigitizerGlobals.vi" "Digitizer Settings"(w5) -> ()
